vi "Set MaxTorque.vi"(8 "error in (no error)":errorcluster, 11 "Value":sgl=9.0) -> (0 "error out":errorcluster)   [LabVIEW 2020, in "输出轴伺服.lvlib"]
uses:
  Servo_global.vi
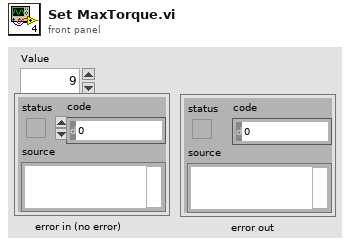
[diagram p1: front panel]
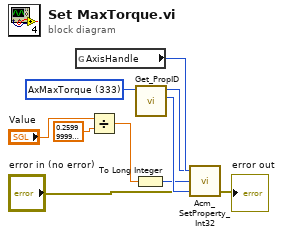
[diagram p0: block diagram]
diagram:
  w8 = u16 333 items=["AxTargetPosition"=44, "AxTargetVelocity"=45, "AxTargetTorque"=46, "AxControlWord"=47, "AxStatusWord"=48, "AxOperationMode"=49, "AxMaxTorque"=333] ("Prop")
  n1 = global read "Servo_global.vi" "AxisHandle"() -> (w10:u32)
  n2 = Divide(x="Value", y=sgl 0.26) -> (x/y=w2:sgl)
  n3 = To Long Integer(number=w2) -> (32bit integer=w1:i32)
  n4 = call "Get_PropID.vi"("Prop"=w8) -> ("BufferLength"=w7:u32, "PropID"=w9:u32)  [unwired: 9 in]
  n5 = call <userlib>:"Acm_SetProperty_Int32.vi"("Handle"=w10, "ProperyID"=w9, "Buffer"=w1, "Error Input(No Error)"="error in (no error)", "BufferLength"=w7) -> ("Error Output"=→"error out":errorcluster)  [unwired: 2 out]
